vi "Get Channel Count.vi"(11 "variant in":variant) -> (1 "number of channels":i32, 3 "variant out":variant)   [LabVIEW 2017]
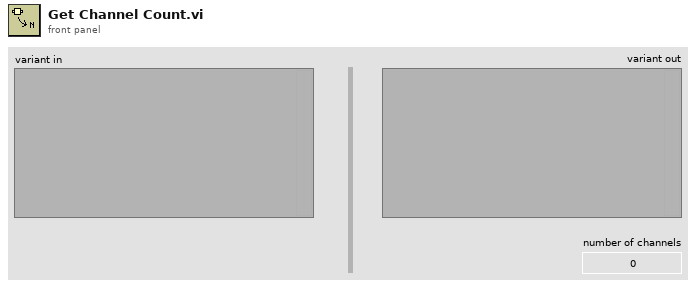
[diagram p1: front panel]
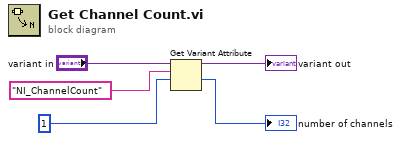
[diagram p0: block diagram]
diagram:
  n1 = Get Variant Attribute(Variant="variant in", name="NI_ChannelCount" ("TDMS property name"), default value (empty Variant)=1 ("timestamp")) -> (duplicate Variant=→"variant out":variant, value=→"number of channels":i32)  [unwired: 1 in, 2 out]
